vi "ConfigureClk.vi"(8 "error in (no error)":errorcluster, 10 "ClkName":string, 11 "PXI_MultiTrig in":refnum<class "PXI_MultiTrig.lvclass">) -> (0 "error out":errorcluster, 3 "PXI_MultiTrig out":refnum<class "PXI_MultiTrig.lvclass">)   [LabVIEW 2014, in "SyncPlugins.lvlib" / "PXI_MultiTrig.lvclass"]
uses:
  PXI_MultiTrig.lvclass
  PXI_MultiTrig.lvclass/PXI_MultiTrig.ctl
  Accessors/Read TimingSession.vi
  Accessors/Write TimingSession.vi
  Accessors/Write Clocks.vi
  Accessors/Read RefClkSession.vi
  Accessors/Write RefClkSession.vi
  Accessors/Read Clocks.vi
  <vilib>/Utility/error.llb/Error Cluster From Error Code.vi
  <instrlib>/niSync/niSync.llb/niSync Create Clock (Frequency).vi
  <vilib>/ErrorRing/Error Ring.xnode
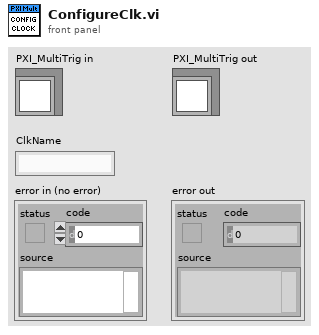
[diagram p1: front panel]
types:
  T1 = typedef "SyncPlugins.lvlib/PXI_MultiTrig.lvclass/clClocks.ctl" = cluster{"Name":string, "RefClk":string, "ClkTerminal":string, "Frequency":dbl, "DutyCycle":dbl, "ClkType":string, "Initiated":bool, "TrigTime":bool}
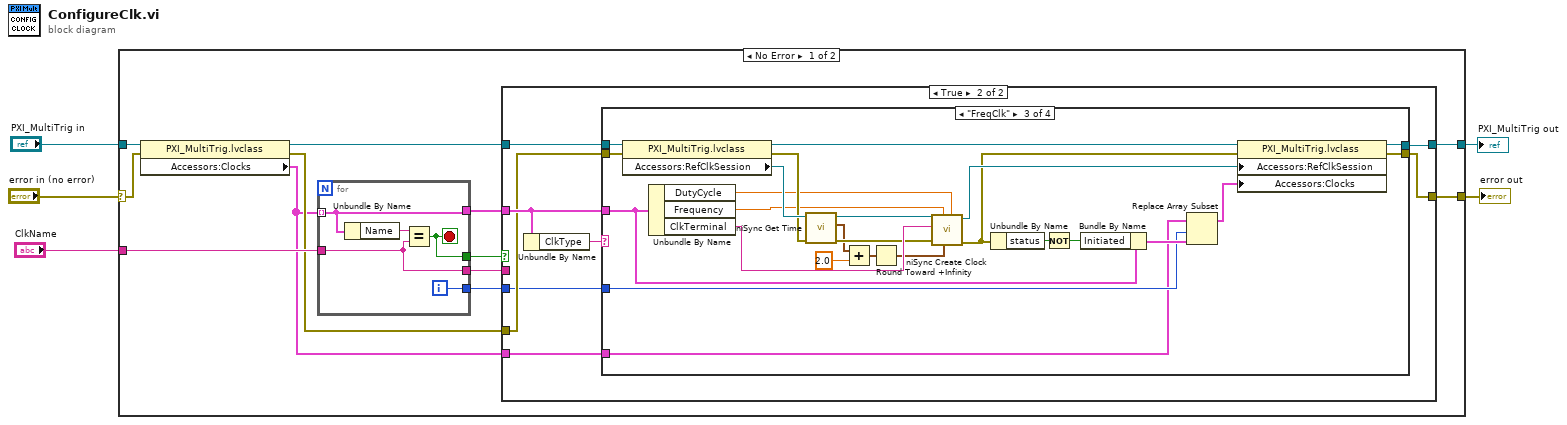
[diagram p0: block diagram]
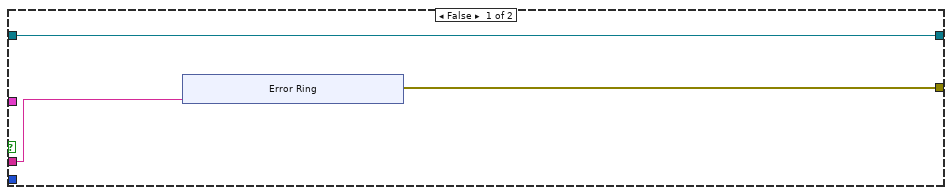
[diagram p2: hidden frame]
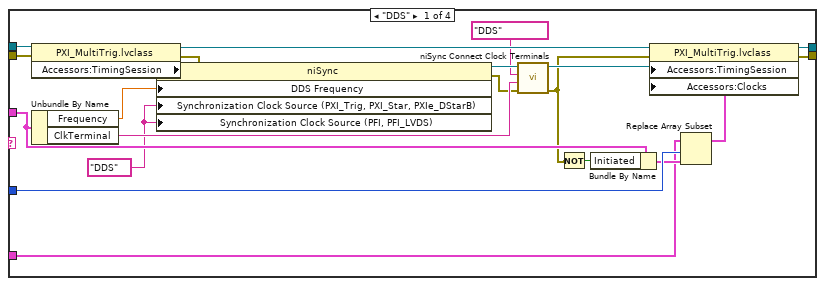
[diagram p3: hidden frame]
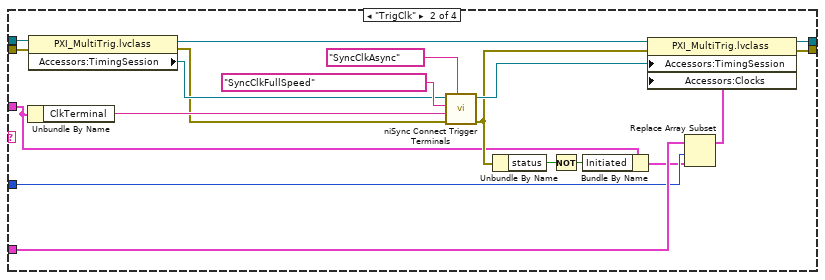
[diagram p4: hidden frame]
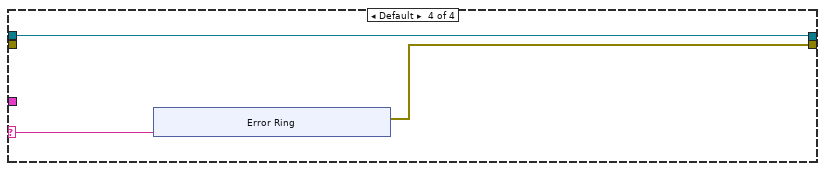
[diagram p5: hidden frame]
diagram:
  n1 = case shown="No Error" "error in (no error)" {
    selector: "error in (no error)" -> [w16 w117]
    tunnel: [w8 w117] -> w4
    tunnel: [w9 w116] -> w2
    tunnel: "PXI_MultiTrig in" -> [w17 w116]
    tunnel: "ClkName" -> [w15 _]
    frame No Error {
      n2 = property class="PXI_MultiTrig.lvclass"(reference=w17, error in=w16) -> (reference out=w10:refnum<class "PXI_MultiTrig.lvclass">, error out=w13:errorcluster, "Accessors:Clocks"=w6:T1[])
      n3 = for {
        tunnel: w6 -> [w114] mode=indexing
        tunnel: w15 -> [w112]
        tunnel: [w114] -> w11
        tunnel: [w113] -> w14
        tunnel: [w112] -> w12
        tunnel: [w111] -> w7
        i -> [w111]
        stop <- w113 stop-if-true
        n4 = Unbundle By Name(w114) -> ("Name"=w115:string)
        n5 = Equal?(x=w115, y=w112) -> (x = y?=w113:bool)
      }
      n6 = case shown="True" w14 {
        tunnel: w13 -> [_ w32]
        tunnel: w12 -> [w20 _]
        tunnel: w11 -> [_ w34]
        tunnel: w10 -> [w19 w33]
        tunnel: [w19 w31] -> w9
        tunnel: [w18 w30] -> w8
        tunnel: w7 -> [_ w29]
        tunnel: w6 -> [_ w28]
        frame False {
          n7 = xnode "Error Ring"("parameter 0"=w20) -> ("error out"=w18:errorcluster)
        }
        frame True {
          n8 = Unbundle By Name(w34) -> ("ClkType"=w35:string)
          n9 = case shown="\"FreqClk\"" w35 {
            selector: w35 -> [_ _ _ w103]
            tunnel: w34 -> [w47 w58 w88 _]
            tunnel: w32 -> [w54 w71 w99 _]
            tunnel: [w49 w67 w98 w102] -> w30
            tunnel: w33 -> [w55 w72 w100 w101]
            tunnel: [w50 w68 w97 w101] -> w31
            tunnel: w29 -> [w46 w60 w90 _]
            tunnel: w28 -> [w44 w61 w89 _]
            frame "DDS" {
              w36 = "DDS" ("Synchronization Clock Properties:Synchronization Clock Source (PXI_Trig, PXI_Star, PXIe_DStarB)")
              n10 = property class="PXI_MultiTrig.lvclass"(reference=w55, error in=w54) -> (reference out=w51:refnum<class "PXI_MultiTrig.lvclass">, error out=w52:errorcluster, "Accessors:TimingSession"=w53:refnum<k15>)
              n11 = Unbundle By Name(w47) -> ("Frequency"=w56:dbl, "ClkTerminal"=w40:string)
              n12 = property class="niSync"(reference=w53, error in=w52, "DDS Frequency"=w56, "Synchronization Clock Source (PXI_Trig, PXI_Star, PXIe_DStarB)"=w36, "Synchronization Clock Source (PFI, PFI_LVDS)"=w36) -> (reference out=w42:refnum<k15>, error out=w39:errorcluster)
              n13 = call <instrlib>:"niSync Connect Clock Terminals.vi"("error in (no error)"=w39, "destination terminal"=w40, "source terminal"="DDS", "instrument handle"=w42) -> ("error out"=w37:errorcluster, "instrument handle out"=w38:refnum<k15>)  [unwired: 6 in]
              n14 = Not(x=w37) -> (.not. x?=w48:bool)
              n15 = Bundle By Name(cluster=w47, "Initiated"=w48) -> (w45:T1)
              n16 = Replace Array Subset(array=w44, new element=w45, index=w46) -> (w43:T1[])
              n17 = property class="PXI_MultiTrig.lvclass"(reference=w51, error in=w37, "Accessors:TimingSession"=w38, "Accessors:Clocks"=w43) -> (reference out=w50:refnum<class "PXI_MultiTrig.lvclass">, error out=w49:errorcluster)
            }
            frame "TrigClk" {
              n18 = Unbundle By Name(w58) -> ("ClkTerminal"=w75:string)
              n19 = property class="PXI_MultiTrig.lvclass"(reference=w72, error in=w71) -> (reference out=w66:refnum<class "PXI_MultiTrig.lvclass">, error out=w69:errorcluster, "Accessors:TimingSession"=w70:refnum<k15>)
              n20 = call <instrlib>:"niSync Connect Trigger Terminals.vi"("synchronization clock"="SyncClkAsync", "error in (no error)"=w69, "destination terminal"=w75, "source terminal"="SyncClkFullSpeed", "instrument handle"=w70) -> ("error out"=w62:errorcluster, "instrument handle out"=w65:refnum<k15>)  [unwired: 5 in]
              n21 = Unbundle By Name(w62) -> ("status"=w63:bool)
              n22 = Not(x=w63) -> (.not. x?=w64:bool)
              n23 = Bundle By Name(cluster=w58, "Initiated"=w64) -> (w59:T1)
              n24 = Replace Array Subset(array=w61, new element=w59, index=w60) -> (w57:T1[])
              n25 = property class="PXI_MultiTrig.lvclass"(reference=w66, error in=w62, "Accessors:TimingSession"=w65, "Accessors:Clocks"=w57) -> (reference out=w68:refnum<class "PXI_MultiTrig.lvclass">, error out=w67:errorcluster)
            }
            frame "FreqClk" {
              n26 = property class="PXI_MultiTrig.lvclass"(reference=w100, error in=w99) -> (reference out=w96:refnum<class "PXI_MultiTrig.lvclass">, error out=w83:errorcluster, "Accessors:RefClkSession"=w84:refnum<k15>)
              n27 = Unbundle By Name(w88) -> ("DutyCycle"=w77:dbl, "Frequency"=w76:dbl, "ClkTerminal"=w86:string)
              n28 = call <instrlib>:"niSync Get Time.vi"("error in (no error)"=w83, "instrument handle"=w84) -> ("error out"=w82:errorcluster, "time"=w81:timestamp, "instrument handle out"=w85:refnum<k15>)  [unwired: 5 in]
              n29 = Add(x=w81, y=2.0) -> (x+y=w79:timestamp)
              n30 = Round Toward +Infinity(x=w79) -> (ceil(x): smallest int >= x=w78:timestamp)
              n31 = call-poly <instrlib>:"niSync Create Clock.vi"("duty cycle"=w77, "start time"=w78, "frequency"=w76, "error in (no error)"=w82, "terminal"=w86, "instrument handle"=w85) -> ("error out"=w91:errorcluster, "instrument handle out"=w95:refnum<k15>)  [unwired: 2 in, 2 out]
              n32 = Unbundle By Name(w91) -> ("status"=w93:bool)
              n33 = Not(x=w93) -> (.not. x?=w92:bool)
              n34 = Bundle By Name(cluster=w88, "Initiated"=w92) -> (w94:T1)
              n35 = Replace Array Subset(array=w89, new element=w94, index=w90) -> (w87:T1[])
              n36 = property class="PXI_MultiTrig.lvclass"(reference=w96, error in=w91, "Accessors:RefClkSession"=w95, "Accessors:Clocks"=w87) -> (reference out=w97:refnum<class "PXI_MultiTrig.lvclass">, error out=w98:errorcluster)
            }
            frame Default {
              n37 = xnode "Error Ring"("parameter 0"=w103) -> ("error out"=w102:errorcluster)
            }
          }
        }
      }
    }
    frame Error {
    }
  }
  "error out" <- w4
  "PXI_MultiTrig out" <- w2
